vi "CSTARdll.vi"(8 "error in (no error)":errorcluster, 11 "Inputs":cluster{"t":dbl, "p":dbl, "v":dbl, "z":dbl[]}) -> (0 "error out":errorcluster, 3 "Outputs":T1)   [LabVIEW 2015]
doc: "subroutine CSTARdll(t, p, v, z, cs, ts, ds, ps, ws, ierr, herr, herr_length)\nCalculate the critical flow factor, C*, for nozzle flow of a gas (subroutine was originally named CCRIT).\n\nINPUTS:\nt -- Temperature [K]\np -- Pressure [kPa]\nv -- Vlenum velocity [m/s] (Should generally be set to 0 for calculating stagnation conditions.)\nz -- Composition (array of mole fractions)\n\nOUTPUTS:\ncs -- Critical flow factor [dimensionless]\nts -- Nozzle throat temperature [K]\nds -- Nozzle throat molar density [mol/L]\nps -- Nozzle throat pressure [kPa]\nws -- Nozzle throat speed of sound [m/s]\nierr -- Error flag: 0 - Successful 151 - CSTAR did not converge\nherr -- Error string (character*255 variable)\nherr_length -- length of variable herr (default: 255)"
uses:
  REFPROP.dll
panel:
  # "REFPROP-CSTARdll.vi"
  # "void  CSTARdll(double *t, double *p, double *v, double *z, double *cs, double *ts, double *ds, double *ps, double *ws, int32_t *ierr, CStr herr, int32_t herr_length);"
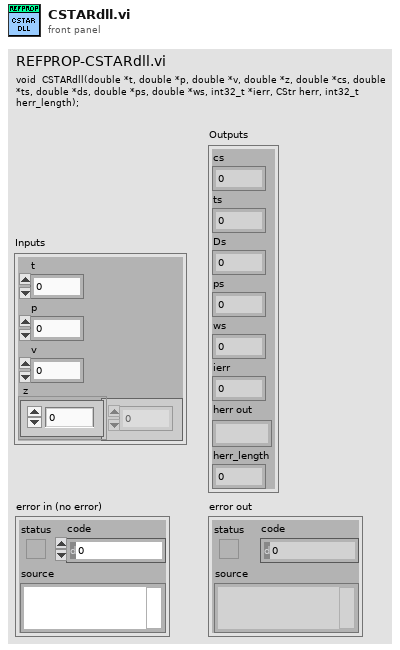
[diagram p1: front panel]
types:
  T1 = cluster{"cs":dbl, "ts":dbl, "Ds":dbl, "ps":dbl, "ws":dbl, "ierr":i32, "herr out":string, "herr_length":i32}
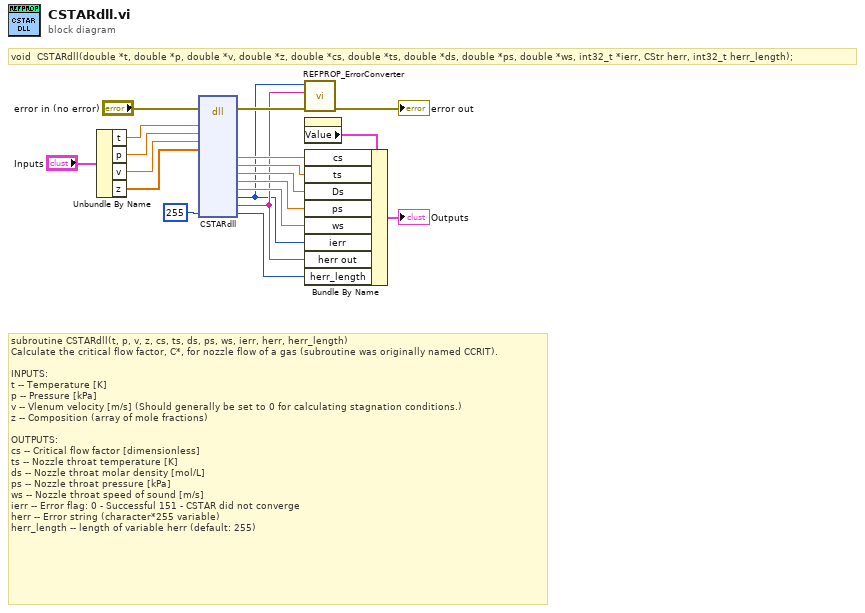
[diagram p0: block diagram]
diagram:
  # "void  CSTARdll(double *t, double *p, double *v, double *z, double *cs, double *ts, double *ds, double *ps, double *ws, int32_t *ierr, CStr herr, int32_t herr_length);"
  # "subroutine CSTARdll(t, p, v, z, cs, ts, ds, ps, ws, ierr, herr, herr_length)\nCalculate the critical flow factor, C*, for nozzle flow of a gas (subroutine was originally named CCRIT).\n\nINPUTS:\nt -- Temperature [K]\np -- Pressure [kPa]\nv -- Vlenum velocity [m/s] (Should generally be set to 0 for calculating stagnation conditions.)\nz -- Composition (array of mole fractions)\n\nOUTPUTS:\ncs -- Critical flow factor [dimensionless]\nts -- Nozzle throat temperature [K]\nds -- Nozzle throat molar density [mol/L]\nps -- Nozzle throat pressure [kPa]\nws -- Nozzle throat speed of sound [m/s]\nierr -- Error flag: 0 - Successful 151 - CSTAR did not converge\nherr -- Error string (character*255 variable)\nherr_length -- length of variable herr (default: 255)"
  n1 = Unbundle By Name("Inputs") -> ("t"=w11:dbl, "p"=w12:dbl, "v"=w13:dbl, "z"=w14:dbl[])
  n2 = dll-call lib="C:/Users/lauria/Desktop/REFPROP 10 LabVIEW Wrapper BETA/REFPROP/REFPROP.*" fn="CSTARdll"(error in="error in (no error)", "t"=w11, "p"=w12, "v"=w13, "z"=w14, "herr_length"=255 ("ln")) -> (error out=w18:errorcluster, "cs"=w3:dbl, "ts"=w4:dbl, "ds"=w5:dbl, "ps"=w6:dbl, "ws"=w7:dbl, "ierr"=w1:i32, "herr"=w2:string, "herr_length"=w8:i32)  [unwired: 14 in, 1 out]
  n3 = call "REFPROP_ErrorConverter.vi"("error in (no error)"=w18, "Error Message"=w2, "Error Code"=w1) -> ("error out"=→"error out":errorcluster)  [unwired: 8 in]
  n4 = property on="Outputs" class="Clust (strict)"() -> ("Value"=w10:T1)  [unwired: 2 in, 2 out]
  n5 = Bundle By Name(cluster=w10, "cs"=w3, "ts"=w4, "Ds"=w5, "ps"=w6, "ws"=w7, "ierr"=w1, "herr out"=w2, "herr_length"=w8) -> (→"Outputs":T1)
